vi "LVClasse_Phase Data addition AB.vi"(0 "Phase in":refnum<class "Phase.lvclass">, 5 "Phase to add":refnum<class "Phase.lvclass">, 11 "error in (no error)":errorcluster) -> (4 "Phase out":refnum<class "Phase.lvclass">, 15 "error out":errorcluster)   [LabVIEW 2020, in "Phase.lvclass"]
doc: "Phase values buffer and pupil setter.\n\n--------------------------------------------------------------------------------\n\n<B>PhaseIn </B> : Phase object.\n<B>PhaseOut </B> : Phase object.\n<B>buffer </B> : Phase values buffer.\n<B>Pupil </B> : pupil object.\n<B>ErrorIn </B> : Error\n<B>ErrorOut </B> : Error\n\n--------------------------------------------------------------------------------"
uses:
  Phase.lvclass
  Phase.lvclass/Phase.ctl
  LVClasse_Phase Read SurfaceFloatWithPupil.vi
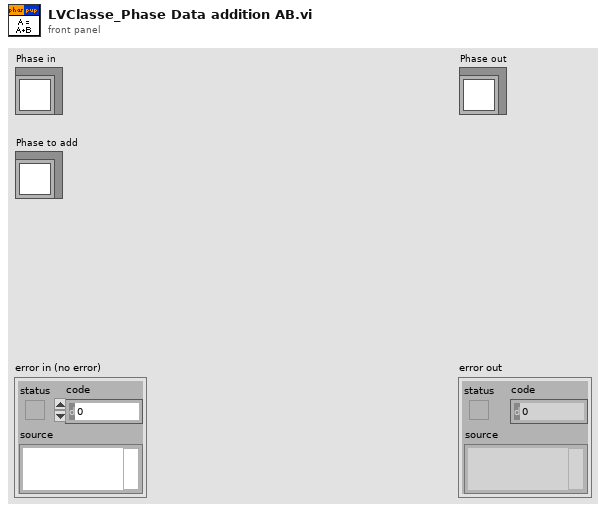
[diagram p1: front panel]
types:
  T1 = typedef "ClassID.ctl" = i64
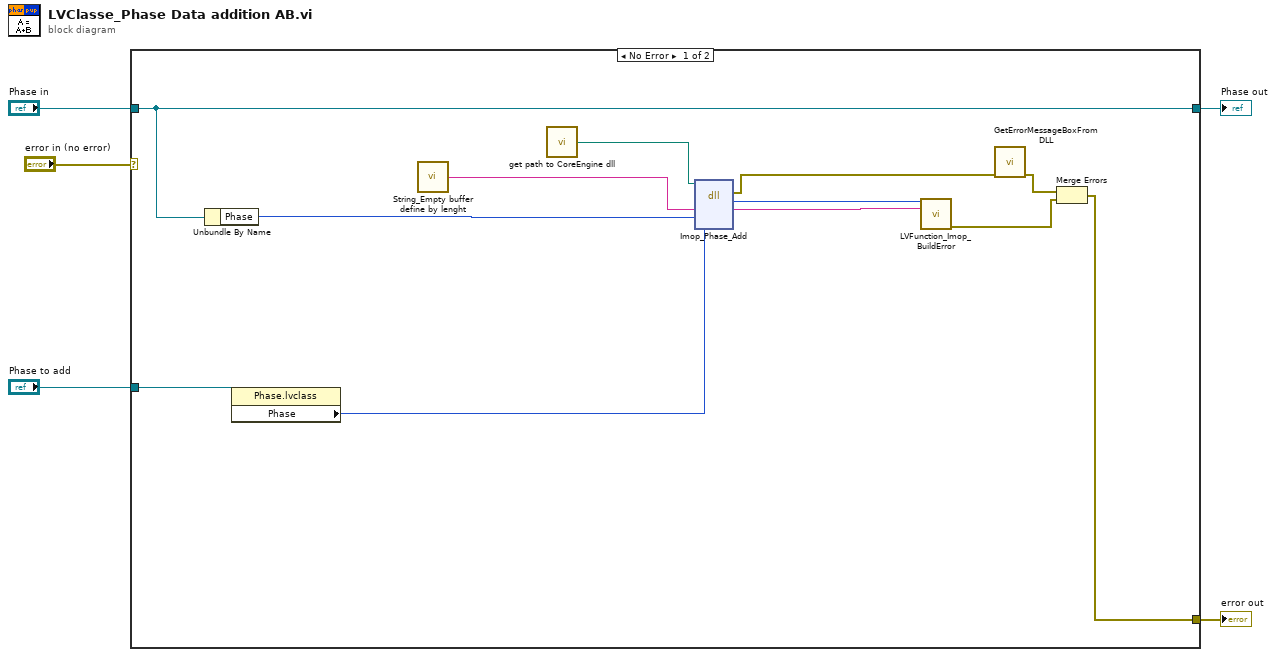
[diagram p0: block diagram]
diagram:
  n1 = case shown="No Error" "error in (no error)" {
    selector: "error in (no error)" -> [_ w19]
    tunnel: [w8 w19] -> w5
    tunnel: [w12 w18] -> w4
    tunnel: "Phase in" -> [w12 w18]
    tunnel: "Phase to add" -> [w7 _]
    frame No Error {
      n2 = Unbundle By Name(w12) -> ("Phase"=w11:T1)
      n3 = property class="Phase.lvclass"(reference=w7) -> ("Phase"=w6:T1)  [unwired: 1 in, 2 out]
      n4 = call "String_Empty buffer define by lenght.vi"() -> ("Empty buffer"=w15:string)  [unwired: 1 in]
      n5 = call "get path to CoreEngine dll.vi"() -> ("path to wavekit library"=w14:path)  [unwired: 14 in, 1 out]
      n6 = dll-call lib="D:/2_trunk/Soft_haso/ImOpCoreEngine4_LV2011/DLLs/ImopEngine4_vc100.dll" fn="Imop_Phase_Add"(path in=w14, "message"=w15, "phase_A"=w11, "phase_B"=w6) -> (error out=w13:errorcluster, "return type"=w17:i32, "message"=w16:string)  [unwired: 4 in, 1 out]
      n7 = call "LVFunction_Imop_BuildError.vi"("code"=w17, "String to Prepend to source (\"\")"=w16) -> ("error out"=w9:errorcluster)  [unwired: 13 in]
      n8 = call "GetErrorMessageBoxFromDLL.vi"("error IN"=w13) -> ("error OUT"=w10:errorcluster)  [unwired: 10 in]
      n9 = Merge Errors(w10, w9) -> (w8:errorcluster)
    }
    frame Error {
    }
  }
  "error out" <- w5
  "Phase out" <- w4
